vi "AsyncWorker.vi"(8 "Error Queue":refnum<queue>, 11 "Command Queue":refnum<queue>) -> ()   [LabVIEW 2015, in "ResultProcessor.lvclass"]
uses:
  ResultProcessor.lvclass
  ErrorQueueDataType.ctl
  Report Information/Report Information.lvclass
  Result/Result.lvclass
  Config/ResultProcessor Config.lvclass
  Report/OnTheFlyReport.lvclass
  Report/Report.lvclass
  CommandQueueDataType.ctl
panel:
  in  "Full Report":T1
  in  "ResultProcessor Config.lvclass":refnum<class "ResultProcessor Config.lvclass">
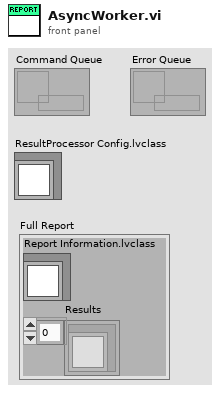
[diagram p1: front panel]
types:
  T1 = cluster{"Report Information.lvclass":refnum<class "Report Information.lvclass">, "Results":refnum<class "Result.lvclass">[]}
  T2 = typedef "ResultProcessor.lvclass/ErrorQueueDataType.ctl" = cluster{"error out":errorcluster}
  T3 = typedef "ResultProcessor.lvclass/CommandQueueDataType.ctl" = cluster{"Command":enum16{"New Report", "Add Result", "Publish Report", "Shutdown", "Add DUT Information", "Add Station Information", "Add Report Information", "Add Test Information"}, "Report Information.lvclass":refnum<class "Report Information.lvclass">, "Result.lvclass":refnum<class "Result.lvclass">}
  T4 = enum16{"New Report", "Add Result", "Publish Report", "Shutdown", "Add DUT Information", "Add Station Information", "Add Report Information", "Add Test Information"}
  T5 = typedef "Report Information.lvclass/DUT Information.ctl" = cluster{"DUT Serial Number":string, "DUT Info":string}
  T6 = typedef "Report Information.lvclass/Station Information.ctl" = cluster{"Station ID":string, "Station Serial Number":string}
  T7 = typedef "Report Information.lvclass/Test Information.ctl" = cluster{"UUT Result":string}
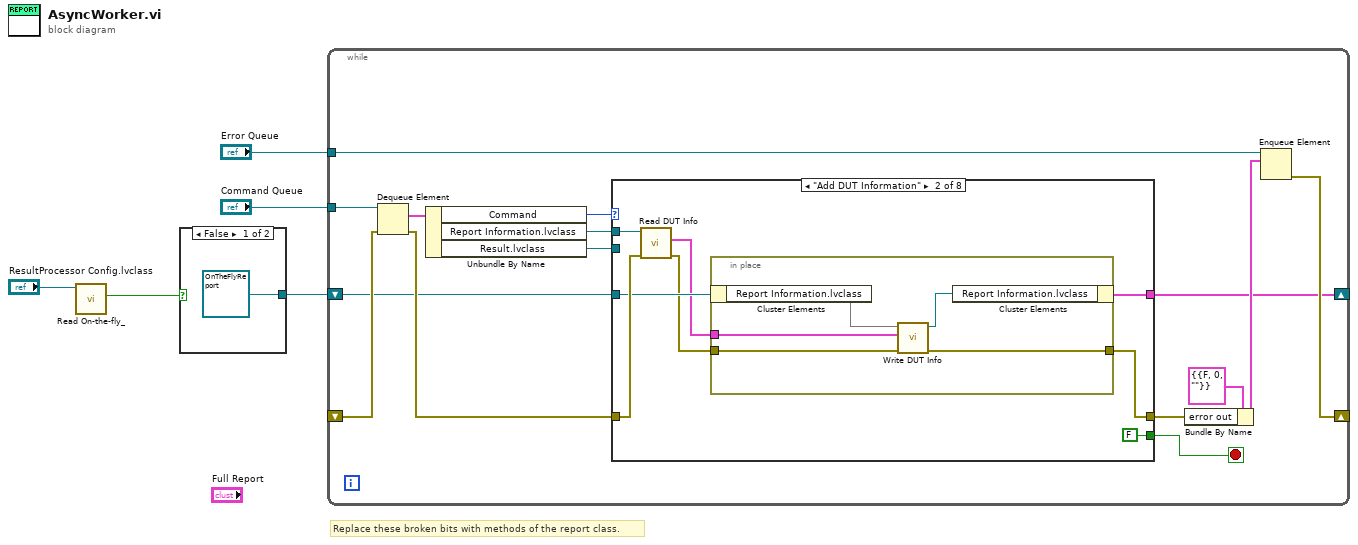
[diagram p0: block diagram]
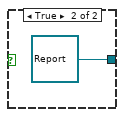
[diagram p2: hidden frame]
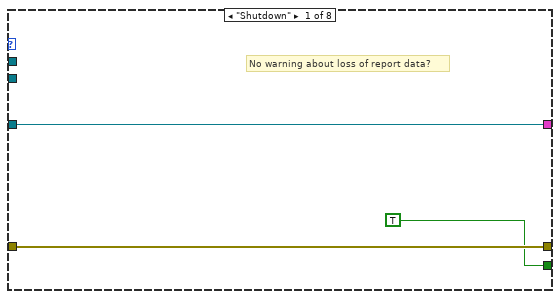
[diagram p3: hidden frame]
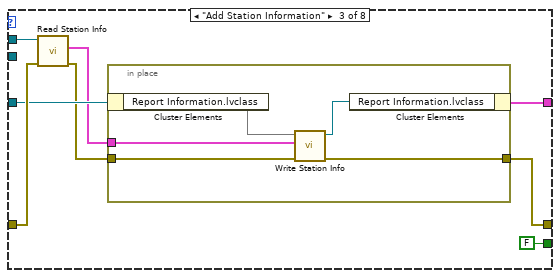
[diagram p4: hidden frame]
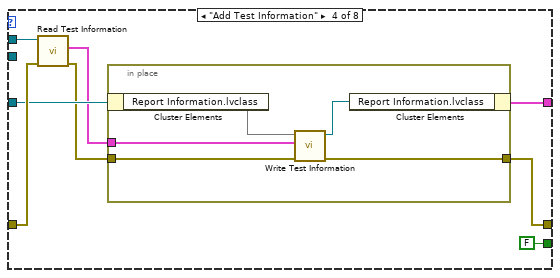
[diagram p5: hidden frame]
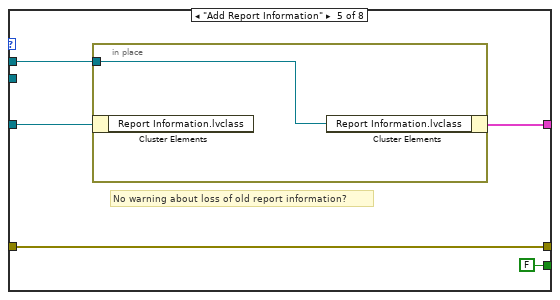
[diagram p6: hidden frame]
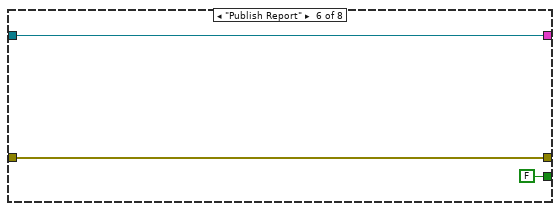
[diagram p7: hidden frame]
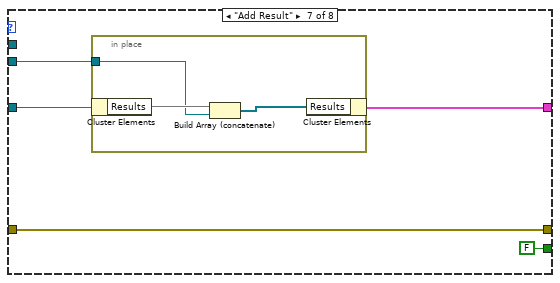
[diagram p8: hidden frame]
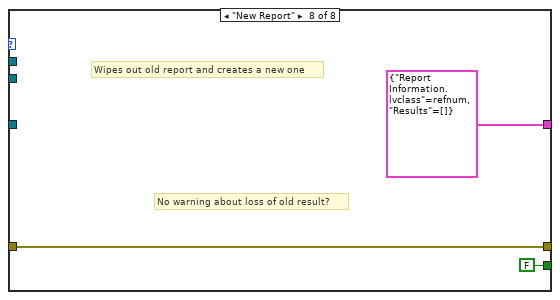
[diagram p9: hidden frame]
diagram:
  # "Replace these broken bits with methods of the report class."
  n1 = call-dynamic "Read On-the-fly_.vi"("ResultProcessor Config in"="ResultProcessor Config.lvclass") -> ("On-the-fly?"=w2:bool)  [unwired: 8 in, 2 out]
  n2 = case shown="False" w2 {
    tunnel: [refnum<class "OnTheFlyReport.lvclass"> refnum ("OnTheFlyReport.lvclass") refnum<class "Report.lvclass"> refnum ("Report.lvclass")] -> w1
    frame False {
    }
    frame True {
    }
  }
  n3 = while {
    tunnel: "Command Queue" -> [w22]
    shift-right: [w15] -> _
    shift-left: _ -> [w20]
    tunnel: "Error Queue" -> [w16]
    shift-right: [w8] -> _
    shift-left: w1 -> [w9]
    stop <- w17 stop-if-true
    n4 = Dequeue Element(queue=w22, error in (no error)=w20) -> (element=w21:T3, error out=w18:errorcluster)  [unwired: 1 in, 2 out]
    n5 = Unbundle By Name(w21) -> ("Command"=w19:T4, "Report Information.lvclass"=w11:refnum<class "Report Information.lvclass">, "Result.lvclass"=w10:refnum<class "Result.lvclass">)
    n6 = case shown="\"Add DUT Information\"" w19 {
      tunnel: w18 -> [w25 w32 w45 w58 w69 w73 w78 w84]
      tunnel: [w25 w28 w41 w54 w69 w73 w78 w84] -> w12
      tunnel: [TRUE FALSE FALSE FALSE FALSE FALSE FALSE FALSE] -> w17
      tunnel: w11 -> [_ w33 w46 w59 w67 _ _ _]
      tunnel: w10 -> [_ _ _ _ _ _ w76 _]
      tunnel: w9 -> [w23 w31 w44 w57 w68 w72 w77 _]
      tunnel: [w23 w27 w40 w53 w66 w72 w75 T1 {"Report Information.lvclass"=refnum, "Results"=[]} ("Full Report")] -> w8
      frame "Shutdown" {
        # "No warning about loss of report data?"
      }
      frame "Add DUT Information" {
        n7 = call-dynamic "Read DUT Info.vi"("error in (no error)"=w32, "Report Information in"=w33) -> ("error out"=w30:errorcluster, "DUT Info"=w29:T5)  [unwired: 7 in, 1 out]
        n8 = in-place {
          in-place-border: w30 -> [w38]
          in-place-border: w29 -> [w37]
          in-place-border: [w34] -> w28
          n9 = in-place-cluster #1(w31) -> ("Report Information.lvclass"=w36)
          n10 = call-dynamic "Write DUT Info.vi"("error in (no error)"=w38, "DUT Info"=w37, "Report Information in"=w36) -> ("error out"=w34:errorcluster, "Report Information out"=w35:refnum<class "Report Information.lvclass">)  [unwired: 7 in]
          n11 = in-place-cluster #1("Report Information.lvclass"=w35) -> (w27:cluster{})
        }
      }
      frame "Add Station Information" {
        n12 = call-dynamic "Read Station Info.vi"("error in (no error)"=w45, "Report Information in"=w46) -> ("error out"=w43:errorcluster, "Station Info"=w42:T6)  [unwired: 7 in, 1 out]
        n13 = in-place {
          in-place-border: w43 -> [w51]
          in-place-border: w42 -> [w50]
          in-place-border: [w47] -> w41
          n14 = in-place-cluster #2(w44) -> ("Report Information.lvclass"=w49)
          n15 = call-dynamic "Write Station Info.vi"("error in (no error)"=w51, "Station Info"=w50, "Report Information in"=w49) -> ("error out"=w47:errorcluster, "Report Information out"=w48:refnum<class "Report Information.lvclass">)  [unwired: 7 in]
          n16 = in-place-cluster #2("Report Information.lvclass"=w48) -> (w40:cluster{})
        }
      }
      frame "Add Test Information" {
        n17 = call-dynamic "Read Test Information.vi"("error in (no error)"=w58, "Report Information in"=w59) -> ("error out"=w56:errorcluster, "Test Information"=w55:T7)  [unwired: 7 in, 1 out]
        n18 = in-place {
          in-place-border: w56 -> [w64]
          in-place-border: w55 -> [w63]
          in-place-border: [w60] -> w54
          n19 = in-place-cluster #3(w57) -> ("Report Information.lvclass"=w62)
          n20 = call-dynamic "Write Test Information.vi"("error in (no error)"=w64, "Test Information"=w63, "Report Information in"=w62) -> ("error out"=w60:errorcluster, "Report Information out"=w61:refnum<class "Report Information.lvclass">)  [unwired: 7 in]
          n21 = in-place-cluster #3("Report Information.lvclass"=w61) -> (w53:cluster{})
        }
      }
      frame "Add Report Information" {
        # "No warning about loss of old report information?"
        n22 = in-place {
          in-place-border: w67 -> [w70]
          n23 = in-place-cluster #4(w68) -> ()  [unwired: 1 out]
          n24 = in-place-cluster #4("Report Information.lvclass"=w70) -> (w66:cluster{})
        }
      }
      frame "Publish Report" {
      }
      frame "Add Result" {
        n25 = in-place {
          in-place-border: w76 -> [w80]
          n26 = in-place-cluster #5(w77) -> ("Results"=w81)
          n27 = Build Array (concatenate)(w81, w80) -> (w79:refnum<class "Result.lvclass">[])
          n28 = in-place-cluster #5("Results"=w79) -> (w75:cluster{})
        }
      }
      frame "New Report" {
        # "No warning about loss of old result?"
        # "Wipes out old report and creates a new one"
      }
    }
    n29 = Bundle By Name(cluster=T2 {"error out"={"status"=FALSE, "code"=0, "source"=""}} ("element"), "error out"=w12) -> (w13:T2)
    n30 = Enqueue Element(queue=w16, element=w13) -> (error out=w15:errorcluster)  [unwired: 2 in, 2 out]
  }
